vi "configure_elo_old.vi"(6 "UVP (Enable)":bool, 9 "Serial Configuration":cluster{"Baud Rate":u32, "Stop Bits":u16}={"Baud Rate"=19200, "Stop Bits"=20} {"Stop Bits" items=["1.0"=10, "2.0"=20]; "Baud Rate" items=["2400"=2400, "4800"=4800, "9600"=9600, "19200"=19200]}, 10 "ELO file":path, 11 "VISA Refnum in":refnum<visa-resource-name>) -> (0 "error out":errorcluster, 1 "Array":dbl[](array[numeric]), 2 "Array size":i32, 3 "VISA Refnum out":refnum<visa-resource-name>)   [LabVIEW 2019]
uses:
  <vilib>/Utility/file.llb/Read Delimited Spreadsheet (DBL).vi
  <instrlib>/Kikusui PLZ 4W Series/Kikusui PLZ 4W Series.lvlib
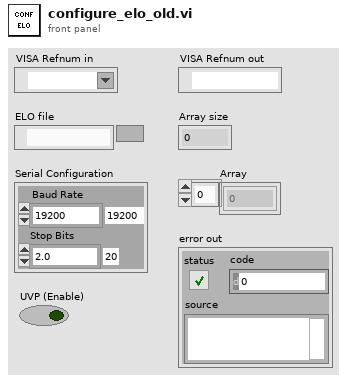
[diagram p1: front panel]
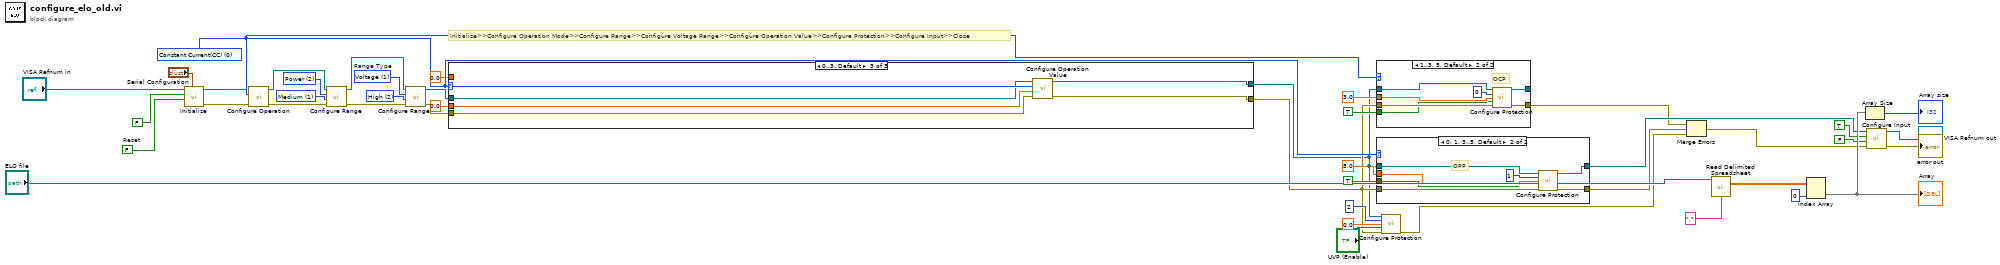
[diagram p0: block diagram]
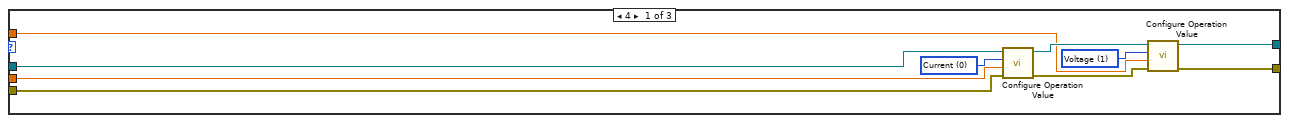
[diagram p4: hidden frame]
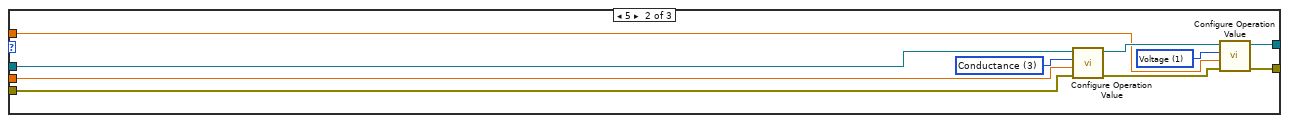
[diagram p5: hidden frame]
diagram:
  w33 = u16 2 items=["Current", "Voltage", "Power", "Conductance"] ("Range Type (0:Current)")
  w13 = u16 2 items=["Low"=0, "High"=2] ("Voltage Range (0:Low)")
  w14 = u16 1 items=["Low", "Medium", "High"] ("Input Range (0:Low)")
  w41 = u16 0 items=["Constant Current(CC)", "Constant Voltage(CV)", "Constant Power(CP)", "Constant Resistance(CR)", "Constant Current & Voltage(CCCV)", "Constant Resistance & Voltage(CRCV)"] ("Operation Mode (0:Constant Current)")
  w29 = FALSE  # Reset
  w12 = u16 1 items=["Current", "Voltage", "Power", "Conductance"]  # Range Type
  # "Initialize>>Configure Operation Mode>>Configure Range>>Configure Voltage Range>>Configure Operation Value>>Configure Protection>>Configure Input>>Close"
  n1 = call <instrlib>:"Initialize.vi"("Serial Configuration"="Serial Configuration", "Reset (True)"=w29, "ID Query (True)"=FALSE, "VISA resource name"="VISA Refnum in") -> ("error out"=w5:errorcluster, "VISA resource name out"=w4:refnum<visa-resource-name>)  [unwired: 6 in]
  n2 = call <instrlib>:"Configure Operation.vi"("error in (no error)"=w5, "Operation Mode (0:Constant Current)"=w41, "VISA resource name"=w4) -> ("error out"=w11:errorcluster, "VISA resource name out"=w10:refnum<visa-resource-name>)  [unwired: 7 in]
  n3 = call <instrlib>:"Configure Range.vi"("error in (no error)"=w11, "Range (0:Low)"=w14, "Range Type (0:Current)"=w33, "VISA resource name"=w10) -> ("error out"=w9:errorcluster, "VISA resource name out"=w8:refnum<visa-resource-name>)  [unwired: 6 in]
  n4 = call <instrlib>:"Configure Range.vi"("error in (no error)"=w9, "Range (0:Low)"=w13, "Range Type (0:Current)"=w12, "VISA resource name"=w8) -> ("error out"=w7:errorcluster, "VISA resource name out"=w6:refnum<visa-resource-name>)  [unwired: 6 in]
  n5 = case shown="0..3, Default" w41 {
    selector: w41 -> [_ _ w66]
    tunnel: 0.0 ("Input Value(0)") -> [w48 w56 w69]
    tunnel: w6 -> [w53 w61 w65]
    tunnel: w7 -> [w52 w60 w64]
    tunnel: [w49 w59 w68] -> w15
    tunnel: [w46 w58 w67] -> w16
    tunnel: 0.0 ("Voltage Value (0)") -> [w47 w57 _]
    frame 4 {
      w44 = u16 1 items=["Current", "Voltage", "Power", "Conductance"] ("Value Type (0:Current)")
      w45 = u16 0 items=["Current", "Voltage", "Power", "Conductance"] ("Value Type (0:Current)")
      n6 = call <instrlib>:"Configure Operation Value.vi"("error in (no error)"=w52, "Values (0)"=w48, "Value Type (0:Current)"=w45, "VISA resource name"=w53) -> ("error out"=w50:errorcluster, "VISA resource name out"=w51:refnum<visa-resource-name>)  [unwired: 6 in]
      n7 = call <instrlib>:"Configure Operation Value.vi"("error in (no error)"=w50, "Values (0)"=w47, "Value Type (0:Current)"=w44, "VISA resource name"=w51) -> ("error out"=w46:errorcluster, "VISA resource name out"=w49:refnum<visa-resource-name>)  [unwired: 6 in]
    }
    frame 5 {
      w54 = u16 1 items=["Current", "Voltage", "Power", "Conductance"] ("Value Type (0:Current)")
      w55 = u16 3 items=["Current", "Voltage", "Power", "Conductance"] ("Value Type (0:Current)")
      n8 = call <instrlib>:"Configure Operation Value.vi"("error in (no error)"=w60, "Values (0)"=w56, "Value Type (0:Current)"=w55, "VISA resource name"=w61) -> ("error out"=w62:errorcluster, "VISA resource name out"=w63:refnum<visa-resource-name>)  [unwired: 6 in]
      n9 = call <instrlib>:"Configure Operation Value.vi"("error in (no error)"=w62, "Values (0)"=w57, "Value Type (0:Current)"=w54, "VISA resource name"=w63) -> ("error out"=w58:errorcluster, "VISA resource name out"=w59:refnum<visa-resource-name>)  [unwired: 6 in]
    }
    frame 0..3, Default {
      n10 = call <instrlib>:"Configure Operation Value.vi"("error in (no error)"=w64, "Values (0)"=w69, "Value Type (0:Current)"=w66, "VISA resource name"=w65) -> ("error out"=w67:errorcluster, "VISA resource name out"=w68:refnum<visa-resource-name>)  [unwired: 6 in]
    }
  }
  n11 = case shown="1..3, 5, Default" w41 {
    tunnel: w15 -> [w71 w78]
    tunnel: w16 -> [w70 w77]
    tunnel: [w71 w76] -> _
    tunnel: [w70 w75] -> w17
    tunnel: 3.0 ("OCP Limit (0)") -> [_ w74]
    tunnel: TRUE ("OCP Trip (Disable)") -> [_ w72]
    frame 0, 4 {
    }
    frame 1..3, 5, Default {
      # "OCP"
      n12 = call <instrlib>:"Configure Protection.vi"("VISA resource name"=w78, "Protection Type (0:OCP)"=0, "Protection Limit (0)"=w74, "Enable Trip (Disable)"=w72, "error in (no error)"=w77) -> ("VISA resource name out"=w76:refnum<visa-resource-name>, "error out"=w75:errorcluster)  [unwired: 9 in]
    }
  }
  n13 = case shown="0, 1, 3..5, Default" w41 {
    tunnel: w15 -> [w80 w87]
    tunnel: w16 -> [w79 w86]
    tunnel: [w80 w85] -> w20
    tunnel: [w79 w84] -> w27
    tunnel: 5.0 ("OPP Limit (0)") -> [_ w83]
    tunnel: TRUE ("OPP Trip (Disable)") -> [_ w81]
    frame 2 {
    }
    frame 0, 1, 3..5, Default {
      # "OPP"
      n14 = call <instrlib>:"Configure Protection.vi"("VISA resource name"=w87, "Protection Type (0:OCP)"=1, "Protection Limit (0)"=w83, "Enable Trip (Disable)"=w81, "error in (no error)"=w86) -> ("VISA resource name out"=w85:refnum<visa-resource-name>, "error out"=w84:errorcluster)  [unwired: 9 in]
    }
  }
  n15 = call <instrlib>:"Configure Protection.vi"("VISA resource name"=w15, "Protection Type (0:OCP)"=2, "Protection Limit (0)"=0.0 ("UVP Limit (0)"), "Enable Trip (Disable)"="UVP (Enable)", "error in (no error)"=w16) -> ("error out"=w18:errorcluster)  [unwired: 9 in, 1 out]
  n16 = Merge Errors(w17, w27, w18) -> (w19:errorcluster)
  n17 = call-poly <vilib>:"Read Delimited Spreadsheet.vi"("file path (dialog if empty)"="ELO file", "delimiter (\\t)"="," ("delimiter (\\t)")) -> ("all rows"=w38:dbl[][])  [unwired: 8 in, 5 out]
  n18 = Index Array(array=w38, index (col)=0 ("disabled index (col)")) -> (element=w42:dbl[])  [unwired: 1 in]
  "Array" <- w42
  n19 = Array Size(array=w42) -> (size(s)=→"Array size":i32)
  n20 = call <instrlib>:"Configure Input.vi"("error in (no error)"=w19, "Enable Input Short (Disable)"=FALSE, "Enable Input (Enable)"=TRUE, "VISA resource name"=w20) -> ("error out"=→"error out":errorcluster, "VISA resource name out"=→"VISA Refnum out":refnum<visa-resource-name>)  [unwired: 6 in]
